vi "Set TDMS File Target Properties.vi"(8 "error in (no error)":errorcluster, 10 "Log File Properties":T1, 11 "Refnum in":refnum<k34>) -> (0 "error out":errorcluster, 3 "Refnum out":refnum<k34>)   [LabVIEW 2019, in "Telemetry Engine.lvlib"]
uses:
  Telemetry Engine.lvlib
  Types/Log File Properties.ctl
  Shared/Constants.vi
  Shared/Telemetry Shared.lvlib
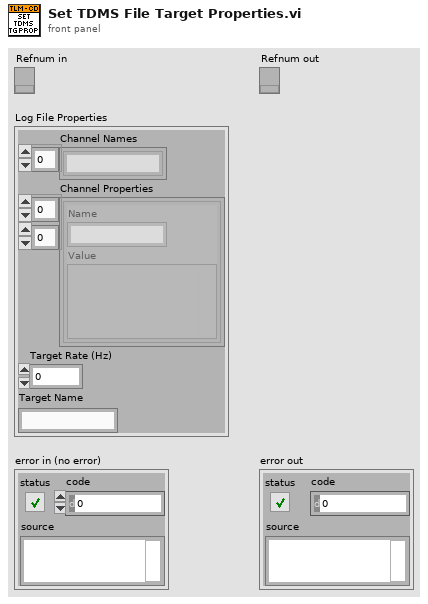
[diagram p1: front panel]
types:
  T1 = typedef "Telemetry Engine.lvlib/Log File Properties.ctl" = cluster{"Channel Names":string[], "Channel Properties":cluster{"Name":string, "Value":variant}[][], "Target Rate (Hz)":dbl, "Target Name":string}
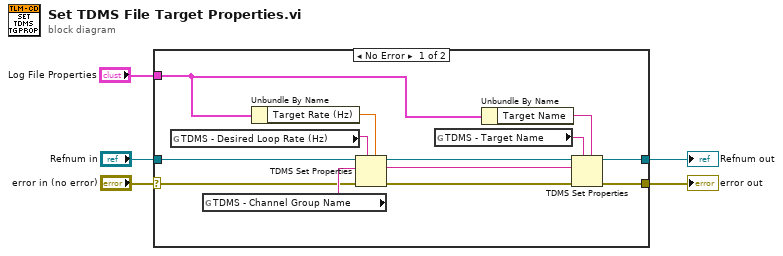
[diagram p0: block diagram]
diagram:
  n1 = case shown="No Error" "error in (no error)" {
    selector: "error in (no error)" -> [w15 w20]
    tunnel: "Log File Properties" -> [w11 _]
    tunnel: "Refnum in" -> [w17 w19]
    tunnel: [w9 w19] -> w3
    tunnel: [w13 w20] -> w2
    frame No Error {
      n2 = global read "Constants.vi" "TDMS - Desired Loop Rate (Hz)"() -> (w8:string)
      n3 = global read "Constants.vi" "TDMS - Channel Group Name"() -> (w16:string)
      n4 = Unbundle By Name(w11) -> ("Target Rate (Hz)"=w18:dbl)
      n5 = TDMS Set Properties(5:w18, 7:w8, 8:w15, 10:w16, 11:w17) -> (0:w14:errorcluster, 2:w12:string, 3:w6:refnum<k34>)  [unwired: 1 in, 1 out]
      n6 = global read "Constants.vi" "TDMS - Target Name"() -> (w7:string)
      n7 = Unbundle By Name(w11) -> ("Target Name"=w10:string)
      n8 = TDMS Set Properties(5:w10, 7:w7, 8:w14, 10:w12, 11:w6) -> (0:w13:errorcluster, 3:w9:refnum<k34>)  [unwired: 1 in, 2 out]
    }
    frame Error {
    }
  }
  "Refnum out" <- w3
  "error out" <- w2
